vi "Main axis motion_單步.vi"(0 "Tacc/Tdec":u32, 1 "axis":u8, 2 "VL/VH":i32, 3 "Position":i32, 4 "¶bemg+":i32, 5 "¶bemg -":i32, 6 "Axis motion function":T1, 7 "error in (no error)":errorcluster, 8 "CK mode":enum16{"motion status", "current position"}(ring), 9 "Ref. data":refnum<vi>, 11 "是否要看軟體極限?":bool) -> (15 "error_code":u32, 17 "current_posi":i32, 19 "error out":errorcluster)   [LabVIEW 2014]
uses:
  axis motion function.ctl
panel:
  in  "error in (no error) 2":errorcluster
  in  "Cluster":T2
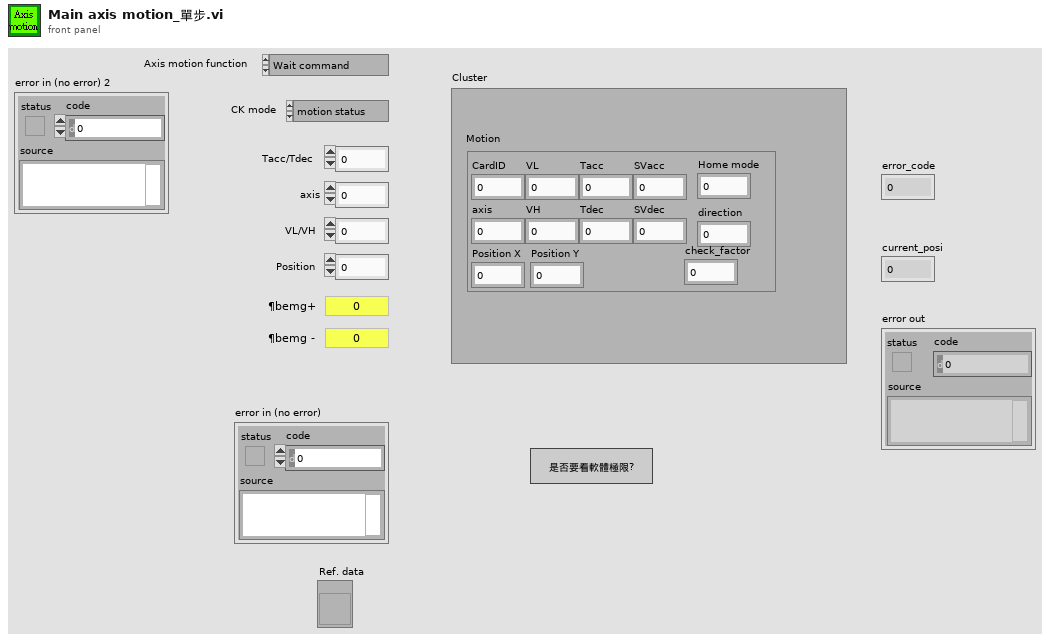
[diagram p1: front panel]
types:
  T1 = typedef "axis motion function.ctl" = enum16{"Wait command", "Axis_S motion", "Axis_P motion", "Axis_Motion_Satus_CK", "Axis _S position CK", "Axis_P position CK", "finish", "error"}
  T2 = cluster{"Motion":cluster{"CardID":u8, "axis":u8, "VL":i32, "VH":i32, "Tacc":u32, "Tdec":u32, "SVacc":u32, "SVdec":u32, "Position X":i32, "Position Y":i32, "Home mode":u8, "direction":u8, "check_factor":u8}}
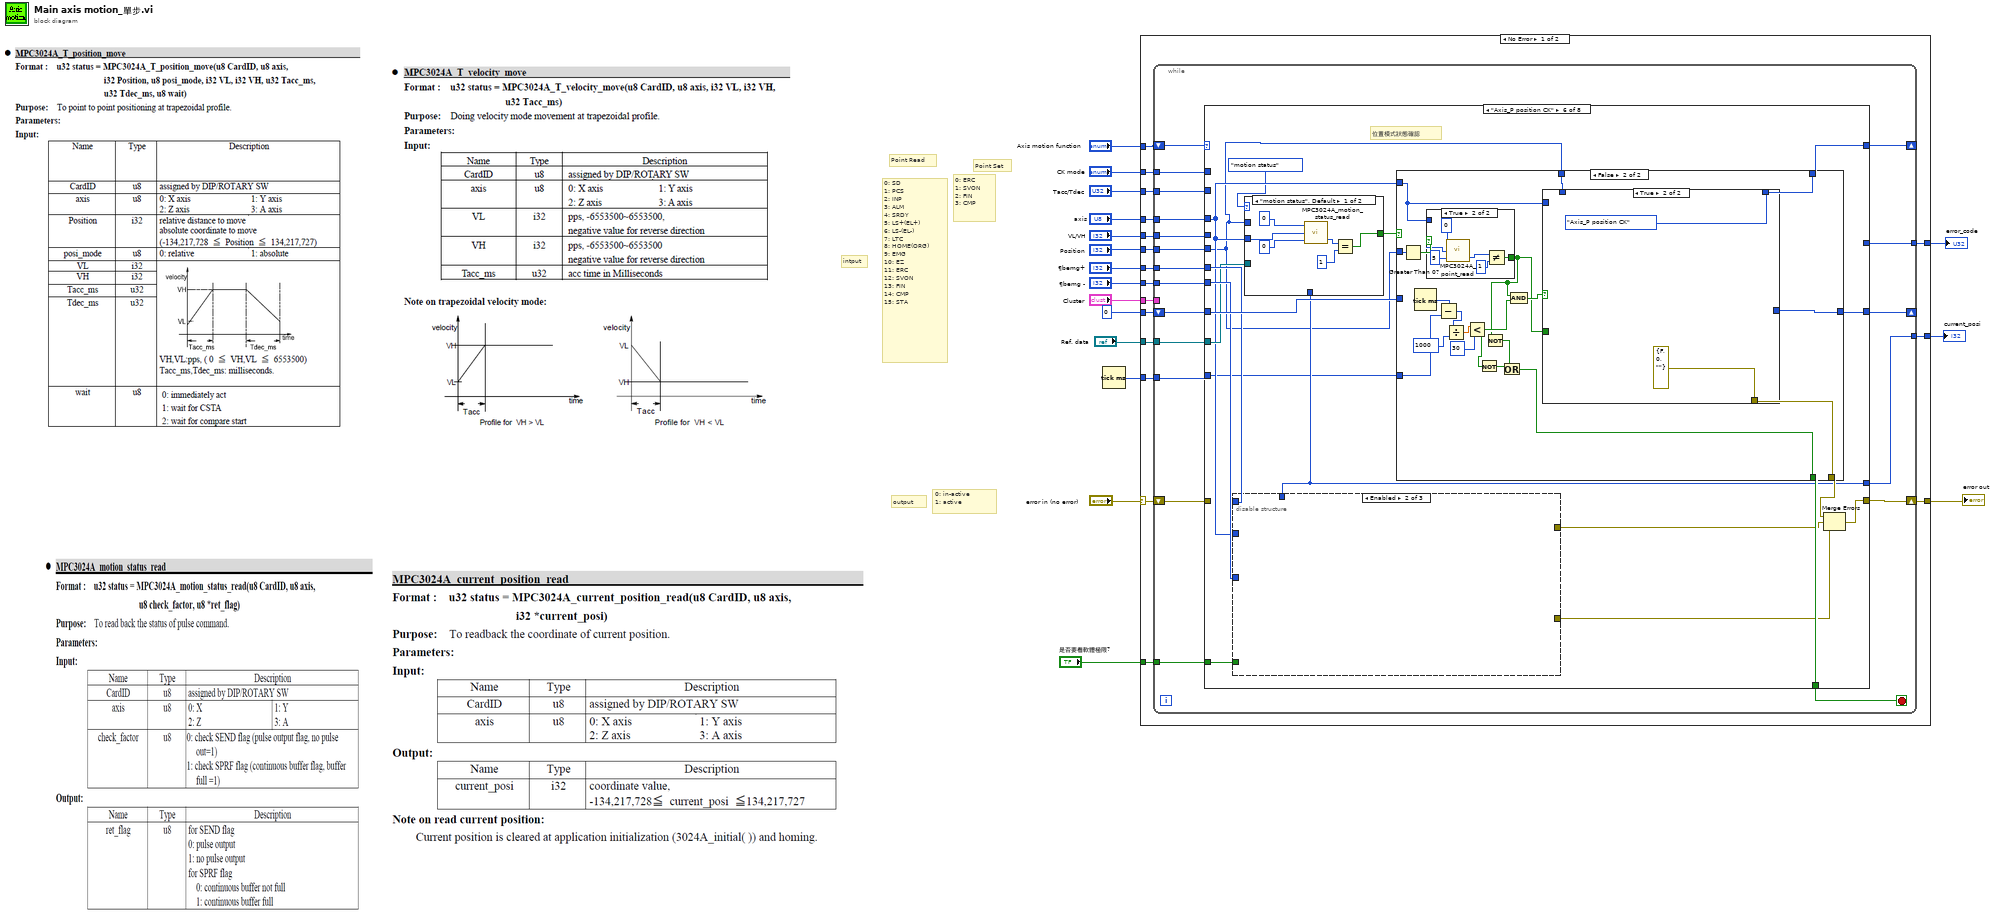
[diagram p0: block diagram]
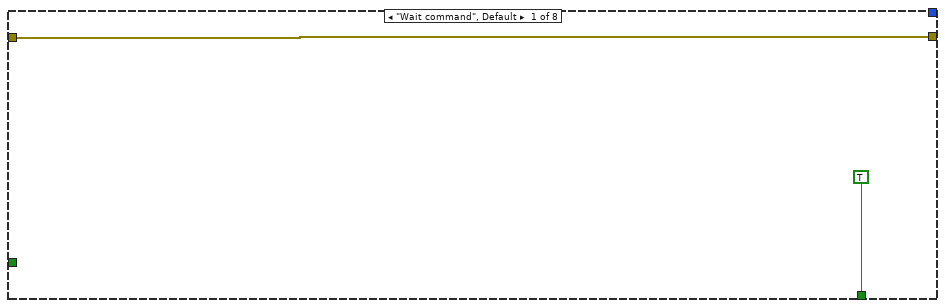
[diagram p2: hidden frame]
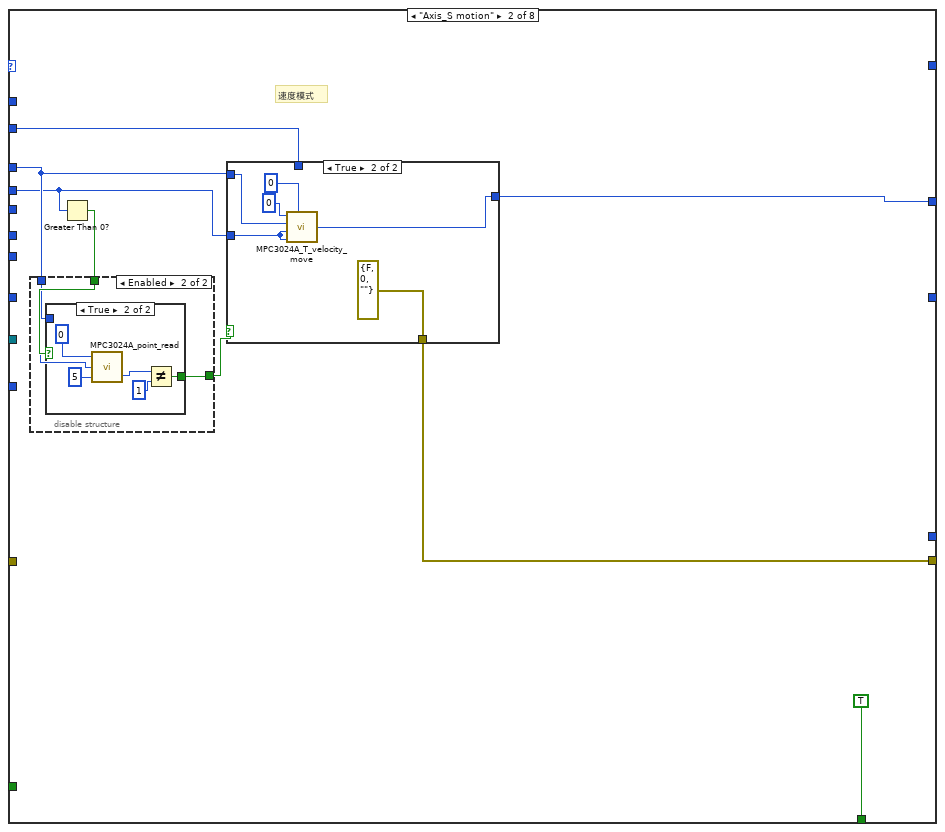
[diagram p3: hidden frame]
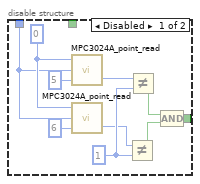
[diagram p4: hidden frame]
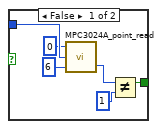
[diagram p5: hidden frame]
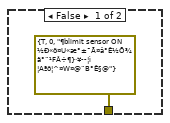
[diagram p6: hidden frame]
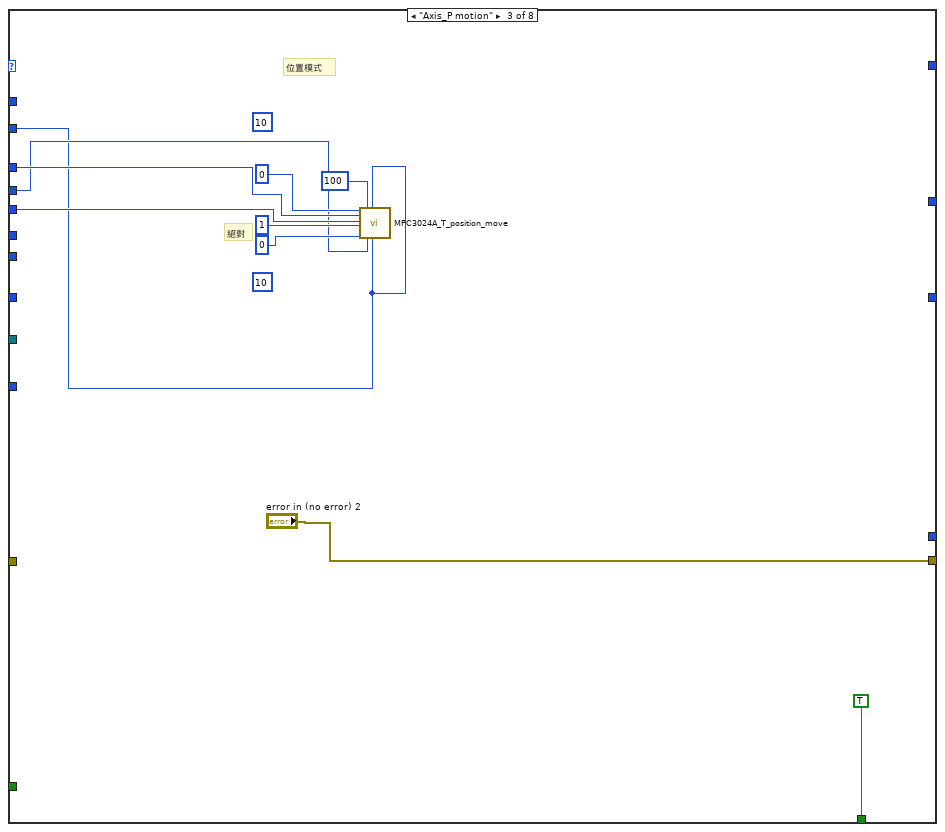
[diagram p7: hidden frame]
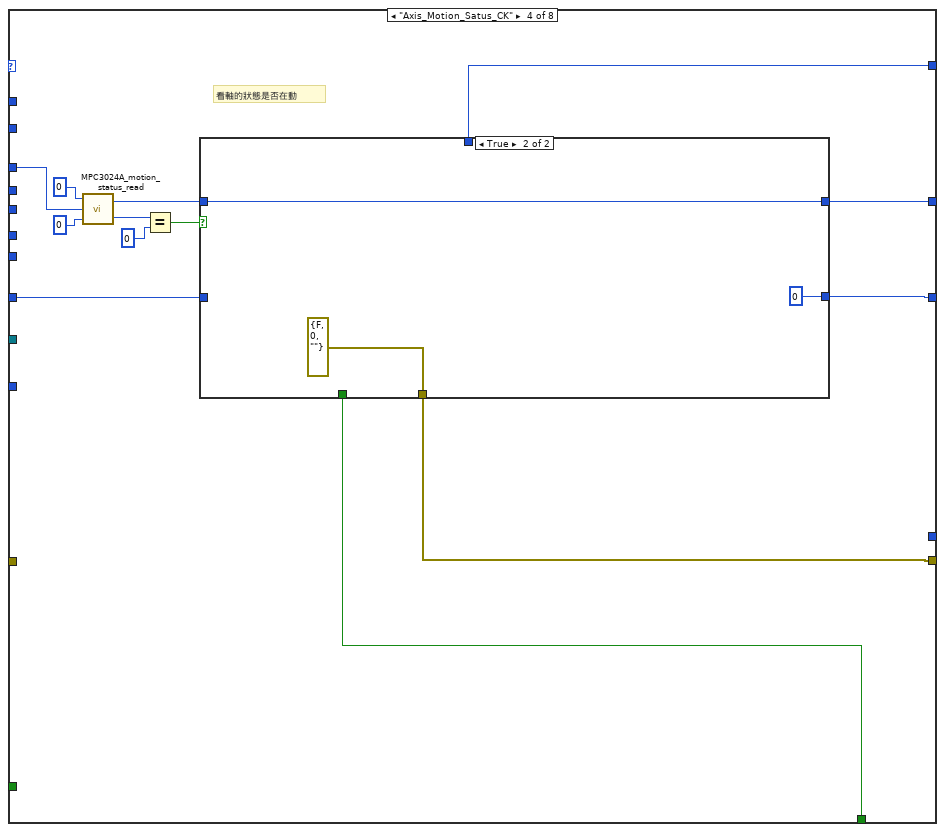
[diagram p8: hidden frame]
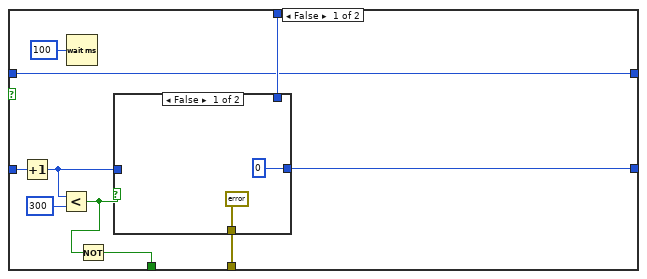
[diagram p9: hidden frame]
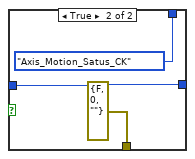
[diagram p10: hidden frame]
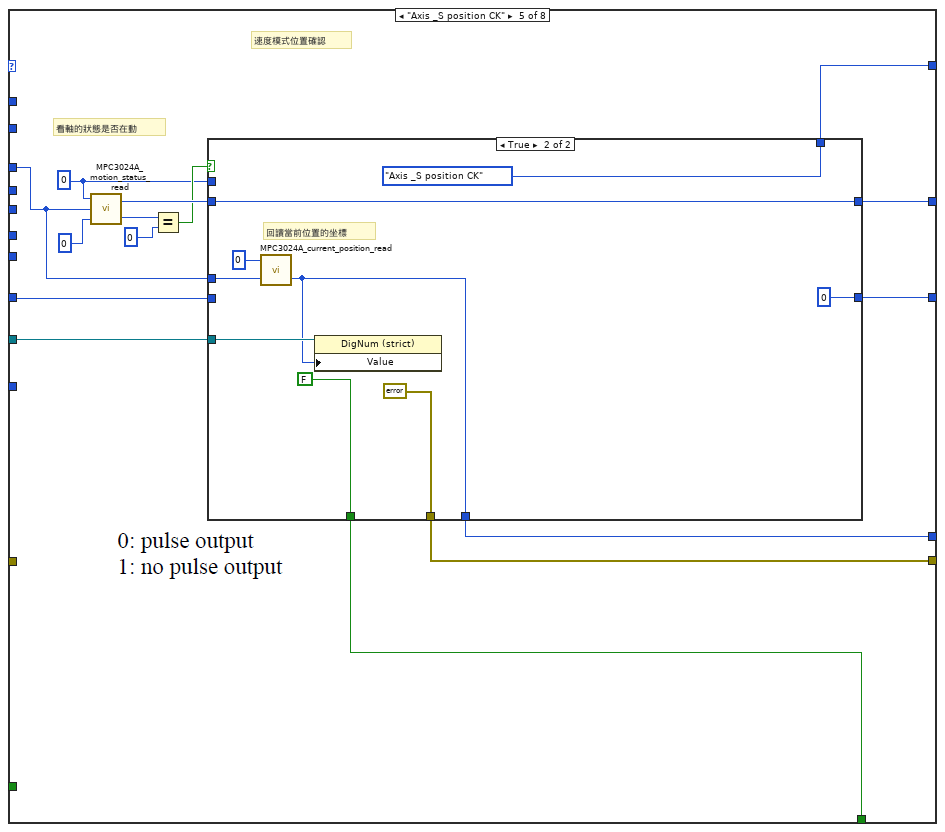
[diagram p11: hidden frame]
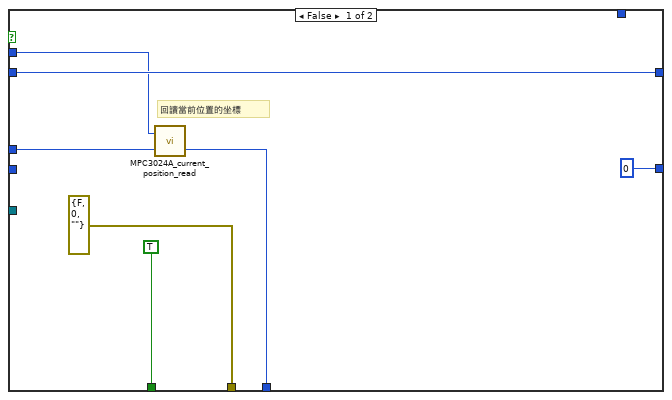
[diagram p12: hidden frame]
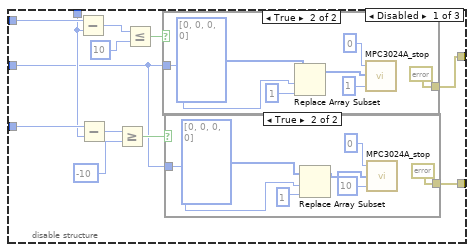
[diagram p13: hidden frame]
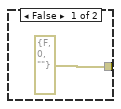
[diagram p14: hidden frame]
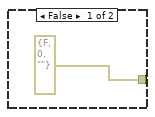
[diagram p15: hidden frame]
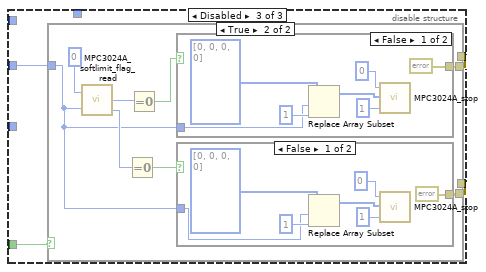
[diagram p16: hidden frame]
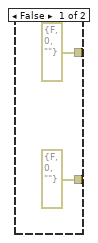
[diagram p17: hidden frame]
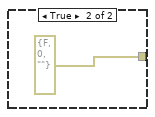
[diagram p18: hidden frame]
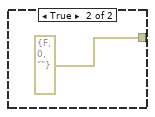
[diagram p19: hidden frame]
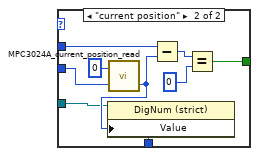
[diagram p20: hidden frame]
diagram:
  # "0: in-active   \n1: active"
  # "output"
  # "intput"
  # "Point Set"
  # "0: ERC   \n1: SVON  \n2: FIN\n3: CMP"
  # "Point Read"
  # "0: SD   \n1: PCS  \n2: INP\n3: ALM\n4: SRDY\n5: LS+(EL+)\n6: LS-(EL-)\n7: LTC\n8: HOME(ORG)\n9: EMG\n10: EZ\n11: ERC\n12: SVON\n13: FIN\n14: CMP\n15: STA"
  n1 = Tick Count (ms)() -> (millisecond timer value=w1:u32)
  n2 = case shown="No Error" "error in (no error)" {
    selector: "error in (no error)" -> [w33 w325]
    tunnel: "Axis motion function" -> [w31 _]
    tunnel: [w34 w325] -> w17
    tunnel: 0 -> [w26 _]
    tunnel: "Cluster" -> [w32 _]
    tunnel: "axis" -> [w30 _]
    tunnel: "VL/VH" -> [w29 _]
    tunnel: "Position" -> [w28 _]
    tunnel: "Tacc/Tdec" -> [w27 _]
    tunnel: [w25 _] -> w8
    tunnel: "CK mode" -> [w24 _]
    tunnel: [w23 _] -> w6
    tunnel: "¶bemg+" -> [w22 _]
    tunnel: "¶bemg -" -> [w21 _]
    tunnel: "Ref. data" -> [w20 _]
    tunnel: "是否要看軟體極限?" -> [w19 _]
    tunnel: w1 -> [w18 _]
    frame No Error {
      n3 = while {
        shift-right: [w45] -> w34
        shift-left: w33 -> [w43]
        tunnel: w32 -> [_]
        shift-right: [w52] -> _
        shift-left: w31 -> [w53]
        tunnel: w30 -> [w51]
        tunnel: w29 -> [w50]
        tunnel: w28 -> [w49]
        tunnel: w27 -> [w48]
        shift-right: [w46] -> _
        shift-left: w26 -> [w47]
        tunnel: [w42] -> w25
        tunnel: w24 -> [w41]
        tunnel: [w40] -> w23
        tunnel: w22 -> [w39]
        tunnel: w21 -> [w38]
        tunnel: w20 -> [w37]
        tunnel: w19 -> [w36]
        tunnel: w18 -> [w35]
        stop <- w44 stop-if-true
        n4 = case shown="\"Axis_P position CK\"" w53 {
          tunnel: [_ _ _ w106 w138 w182 _ _] -> w52
          tunnel: w51 -> [_ w58 w99 w112 w140 w171 _ _]
          tunnel: w50 -> [_ w57 w98 _ _ _ _ _]
          tunnel: w49 -> [_ _ w100 _ _ w168 _ _]
          tunnel: w48 -> [_ w59 w97 _ _ _ _ _]
          tunnel: w47 -> [_ _ _ w109 w150 w185 w320 w323]
          tunnel: [_ _ _ w110 w148 w184 w320 w323] -> w46
          tunnel: [w55 w61 "error in (no error) 2" w108 w151 w179 w321 w324] -> w45
          tunnel: [TRUE TRUE TRUE w111 w149 w183 _ TRUE] -> w44
          tunnel: w43 -> [w55 _ _ _ _ _ w321 w324]
          tunnel: [_ w60 _ w107 w147 _ _ _] -> w42
          tunnel: w41 -> [_ _ _ _ _ _ _ _]
          tunnel: [_ _ _ _ w139 w175 _ _] -> w40
          tunnel: w39 -> [_ _ _ _ _ w180 _ _]
          tunnel: w38 -> [_ _ _ _ _ w176 _ _]
          tunnel: w37 -> [_ _ _ _ w137 w173 _ _]
          tunnel: w36 -> [_ _ _ _ _ w172 _ _]
          tunnel: w35 -> [_ _ _ _ _ w170 _ _]
          frame "Wait command", Default {
          }
          frame "Axis_S motion" {
            # "速度模式"
            n5 = Greater Than 0?(x=w57) -> (x > 0?=w56:bool)
            n6 = disable-structure shown="Enabled" {
              disable-tunnel: [w65 w74] -> w62
              disable-tunnel: w58 -> [w64 w75]
              disable-tunnel: w56 -> [_ w76]
              frame Disabled {
                w66 = u8 0 ("axis")
                w71 = u8 1 ("y")
                n7 = call "MPC3024A_point_read.vi"("check_factor"=u8 5, "axis"=w64, "CardID"=w66) -> ("state"=w70:u8)  [unwired: 1 out]
                n8 = call "MPC3024A_point_read.vi"("check_factor"=u8 6, "axis"=w64, "CardID"=w66) -> ("state"=w69:u8)  [unwired: 1 out]
                n9 = Not Equal?(x=w69, y=w71) -> (x != y?=w68:bool)
                n10 = Not Equal?(x=w70, y=w71) -> (x != y?=w67:bool)
                n11 = Compound Arithmetic op=AND(w67, w68) -> (w65:bool)
              }
              frame Enabled {
                n12 = case shown="True" w76 {
                  tunnel: w75 -> [w81 w86]
                  tunnel: [w77 w83] -> w74
                  frame False {
                    n13 = call "MPC3024A_point_read.vi"("check_factor"=u8 6, "axis"=w81, "CardID"=u8 0) -> ("state"=w78:u8)  [unwired: 1 out]
                    n14 = Not Equal?(x=w78, y=u8 1) -> (x != y?=w77:bool)
                  }
                  frame True {
                    n15 = call "MPC3024A_point_read.vi"("check_factor"=u8 5, "axis"=w86, "CardID"=u8 0 ("axis")) -> ("state"=w85:u8)  [unwired: 1 out]
                    n16 = Not Equal?(x=w85, y=u8 1) -> (x != y?=w83:bool)
                  }
                }
              }
            }
            n17 = case shown="True" w62 {
              tunnel: [_ w95] -> w60
              tunnel: [errorcluster {"status"=TRUE, "code"=0, "source"="¶blimit sensor ON ½Ð«ö¤U«æ°±¯Ã¤â°Ê½Õ¾ã°¨¹FÂ÷¶}·¥­­¦ì ¦Aªð¦^¤W¤@¨B°Ê§@"} ("error in (no error)") errorcluster {"status"=FALSE, "code"=0, "source"=""} ("error in (no error)")] -> w61
              tunnel: w59 -> [_ _]
              tunnel: w58 -> [_ w92]
              tunnel: w57 -> [_ w91]
              frame False {
              }
              frame True {
                n18 = call "MPC3024A_T_velocity_move.vi"("CardID"=u8 0, "axis"=w92, "VL"=w91, "VH"=w91, "Tacc_ms"=u32 0) -> ("error_code"=w95:u32)
              }
            }
          }
          frame "Axis_P motion" {
            (unwired) u32 10 ("Tdec_ms")
            (unwired) u32 10 ("Tacc_ms")
            # "位置模式"
            # "絕對"
            n19 = call "MPC3024A_T_position_move.vi"("CardID"=u8 0, "axis"=w99, "Position"=w100, "posi_mode"=u8 1, "wait"=u8 0, "VL"=100, "VH"=w98, "Tacc_ms"=w97, "Tdec_ms"=w97) -> ()  [unwired: 10 in, 1 out]
          }
          frame "Axis_Motion_Satus_CK" {
            # "看軸的狀態是否在動"
            n20 = call "MPC3024A_motion_status_read.vi"("check_factor"=u8 0, "axis"=w112, "CardID"=u8 0) -> ("ret_fig"=w115:u8, "error_code"=w114:u32)
            n21 = Equal?(x=w115, y=u8 0) -> (x = y?=w113:bool)
            n22 = case shown="True" w113 {
              tunnel: [w124 errorcluster {"status"=FALSE, "code"=0, "source"=""} ("error in (no error)")] -> w108
              tunnel: w109 -> [w119 _]
              tunnel: [w126 _] -> w111
              tunnel: [w123 _] -> w106
              tunnel: [w122 0] -> w110
              tunnel: [w120 w134] -> w107
              tunnel: w114 -> [w120 w134]
              frame False {
                n23 = Increment(x=w119) -> (x+1=w121:i32)
                n24 = Less?(x=w121, y=300) -> (x < y?=w125:bool)
                n25 = Wait (ms)(milliseconds to wait=u32 100) -> ()  [unwired: 1 out]
                n26 = Not(x=w125) -> (.not. x?=w126:bool)
                n27 = case shown="False" w125 {
                  tunnel: [errorcluster {"status"=TRUE, "code"=0, "source"="軸沒輸出移動脈波"} ("error in (no error)") errorcluster {"status"=FALSE, "code"=0, "source"=""} ("error in (no error)")] -> w124
                  tunnel: [_ axis_motion_function."Axis_Motion_Satus_CK" ("Axis motion function")] -> w123
                  tunnel: [0 w131] -> w122
                  tunnel: w121 -> [_ w131]
                  frame False {
                  }
                  frame True {
                  }
                }
              }
              frame True {
              }
            }
          }
          frame "Axis _S position CK" {
            w141 = u8 0 ("CardID")
            # "速度模式位置確認"
            # "看軸的狀態是否在動"
            n28 = call "MPC3024A_motion_status_read.vi"("check_factor"=u8 0, "axis"=w140, "CardID"=w141) -> ("ret_fig"=w144:u8, "error_code"=w143:u32)
            n29 = Equal?(x=w144, y=u8 0) -> (x = y?=w142:bool)
            n30 = case shown="True" w142 {
              tunnel: [errorcluster {"status"=FALSE, "code"=0, "source"=""} ("error in (no error)") errorcluster {"status"=FALSE, "code"=0, "source"=""} ("error in (no error)")] -> w151
              tunnel: w150 -> [_ _]
              tunnel: [TRUE FALSE] -> w149
              tunnel: [_ axis_motion_function."Axis _S position CK" ("Axis motion function")] -> w138
              tunnel: [0 0] -> w148
              tunnel: [w157 w165] -> w147
              tunnel: w143 -> [w157 w165]
              tunnel: w141 -> [w155 _]
              tunnel: w140 -> [w156 w164]
              tunnel: [w152 w161] -> w139
              tunnel: w137 -> [_ w162]
              frame False {
                # "回讀當前位置的坐標"
                n31 = call "MPC3024A_current_position_read.vi"("axis"=w156, "CardID"=w155) -> ("current_posi"=w152:i32)  [unwired: 1 out]
              }
              frame True {
                # "回讀當前位置的坐標"
                n32 = call "MPC3024A_current_position_read.vi"("axis"=w164, "CardID"=u8 0) -> ("current_posi"=w161:i32)  [unwired: 1 out]
                n33 = property class="DigNum (strict)"(reference=w162, "Value"=w161) -> ()  [unwired: 1 in, 2 out]
              }
            }
          }
          frame "Axis_P position CK" {
            # "位置模式狀態確認"
            n34 = case shown="\"motion status\", Default" enum16{"motion status", "current position"}."motion status" ("CK mode") {
              tunnel: [w245 w254] -> w181
              tunnel: w171 -> [w244 w253]
              tunnel: w168 -> [_ w252]
              tunnel: [_ w251] -> w175
              tunnel: w173 -> [_ w250]
              frame "motion status", Default {
                n35 = call "MPC3024A_motion_status_read.vi"("check_factor"=u8 0, "axis"=w244, "CardID"=u8 0) -> ("ret_fig"=w246:u8)  [unwired: 1 out]
                n36 = Equal?(x=w246, y=u8 1) -> (x = y?=w245:bool)
              }
              frame "current position" {
                n37 = call "MPC3024A_current_position_read.vi"("axis"=w253, "CardID"=u8 0) -> ("current_posi"=w251:i32)  [unwired: 1 out]
                n38 = property class="DigNum (strict)"(reference=w250, "Value"=w251) -> ()  [unwired: 1 in, 2 out]
                n39 = Subtract(x=w252, y=w251) -> (x-y=w256:i32)
                n40 = Equal?(x=w256, y=0) -> (x = y?=w254:bool)
              }
            }
            n41 = disable-structure shown="Enabled" {
              disable-tunnel: w180 -> [w197 _ _]
              disable-tunnel: [w193 _ w217] -> w177
              disable-tunnel: w176 -> [w190 _ _]
              disable-tunnel: w175 -> [w189 _ _]
              disable-tunnel: [w188 _ w216] -> w174
              disable-tunnel: w171 -> [w186 _ w214]
              disable-tunnel: w172 -> [_ _ w215]
              frame Disabled {
                n42 = Subtract(x=w197, y=w189) -> (x-y=w196:i32)
                n43 = Subtract(x=w190, y=w189) -> (x-y=w187:i32)
                n44 = Greater Or Equal?(x=w187, y=-10) -> (x >= y?=w192:bool)
                n45 = Less Or Equal?(x=w196, y=10) -> (x <= y?=w194:bool)
                n46 = case shown="True" w194 {
                  tunnel: [errorcluster {"status"=FALSE, "code"=0, "source"=""} ("error in (no error)") errorcluster {"status"=TRUE, "code"=0, "source"="軸接近後軟體極限"} ("error in (no error)")] -> w193
                  tunnel: w186 -> [_ w207]
                  frame False {
                  }
                  frame True {
                    n47 = Replace Array Subset(array=i32[] [0, 0, 0, 0], new element=1 ("new element/subarray"), index=w207) -> (w208:i32[])
                    n48 = call "MPC3024A_stop.vi"("Tdec_ms"=u32 1, "axis[4]"=w208, "CardID"=u8 0) -> ()  [unwired: 1 out]
                  }
                }
                n49 = case shown="True" w192 {
                  tunnel: [errorcluster {"status"=FALSE, "code"=0, "source"=""} ("error in (no error)") errorcluster {"status"=TRUE, "code"=0, "source"="軸接近前軟體極限"} ("error in (no error)")] -> w188
                  tunnel: w186 -> [_ w199]
                  frame False {
                  }
                  frame True {
                    n50 = Replace Array Subset(array=i32[] [0, 0, 0, 0], new element=1 ("new element/subarray"), index=w199) -> (w202:i32[])
                    n51 = call "MPC3024A_stop.vi"("Tdec_ms"=u32 10, "axis[4]"=w202, "CardID"=u8 0) -> ()  [unwired: 1 out]
                  }
                }
              }
              frame Enabled {
              }
              frame Disabled {
                n52 = case shown="True" w215 {
                  tunnel: [errorcluster {"status"=FALSE, "code"=0, "source"=""} ("error in (no error)") w223] -> w217
                  tunnel: [errorcluster {"status"=FALSE, "code"=0, "source"=""} ("error in (no error)") w222] -> w216
                  tunnel: w214 -> [_ w220]
                  frame False {
                  }
                  frame True {
                    n53 = call "MPC3024A_softlimit_flag_read.vi"("CardID"=u8 0, "axis"=w220) -> ("P_limit_flag"=w226:u8, "N_limit_flag"=w225:u8)  [unwired: 1 out]
                    n54 = Equal To 0?(x=w225) -> (x = 0?=w221:bool)
                    n55 = Equal To 0?(x=w226) -> (x = 0?=w224:bool)
                    n56 = case shown="False" w224 {
                      tunnel: [errorcluster {"status"=TRUE, "code"=0, "source"="軸接近前軟體極限"} ("error in (no error)") errorcluster {"status"=FALSE, "code"=0, "source"=""} ("error in (no error)")] -> w223
                      tunnel: w220 -> [w236 _]
                      frame False {
                        n57 = Replace Array Subset(array=i32[] [0, 0, 0, 0], new element=1 ("new element/subarray"), index=w236) -> (w237:i32[])
                        n58 = call "MPC3024A_stop.vi"("Tdec_ms"=u32 1, "axis[4]"=w237, "CardID"=u8 0) -> ()  [unwired: 1 out]
                      }
                      frame True {
                      }
                    }
                    n59 = case shown="False" w221 {
                      tunnel: [errorcluster {"status"=TRUE, "code"=0, "source"="軸接近後軟體極限"} ("error in (no error)") errorcluster {"status"=FALSE, "code"=0, "source"=""} ("error in (no error)")] -> w222
                      tunnel: w220 -> [w228 _]
                      frame False {
                        n60 = Replace Array Subset(array=i32[] [0, 0, 0, 0], new element=1 ("new element/subarray"), index=w228) -> (w229:i32[])
                        n61 = call "MPC3024A_stop.vi"("Tdec_ms"=u32 1, "axis[4]"=w229, "CardID"=u8 0) -> ()  [unwired: 1 out]
                      }
                      frame True {
                      }
                    }
                  }
                }
              }
            }
            n62 = case shown="False" w181 {
              selector: w181 -> [w262 _]
              tunnel: w185 -> [_ _]
              tunnel: [_ w289] -> w184
              tunnel: [w267 w290] -> w178
              tunnel: [w262 w274] -> w183
              tunnel: [axis_motion_function."finish" ("Axis motion function") w291] -> w182
              tunnel: w168 -> [_ w287]
              tunnel: w171 -> [w266 w275]
              tunnel: w170 -> [_ w285]
              tunnel: w168 -> [w265 w279]
              frame True {
                # "+-10pulse"
                n63 = call "MPC3024A_current_position_read.vi"("axis"=w266, "CardID"=u8 0) -> ("current_posi"=w263:i32)  [unwired: 1 out]
                n64 = Subtract(x=w265, y=w263) -> (x-y=w261:i32)
                n65 = In Range and Coerce(upper limit=10.0, x=w261, lower limit=10.0 ("upper limit")) -> (In Range?=w258:bool)  [unwired: 1 out]
                n66 = disable-structure shown="Disabled" {
                  disable-tunnel: [w270 _] -> w267
                  disable-tunnel: w258 -> [w269 _]
                  frame Disabled {
                    n67 = case shown="False" w269 {
                      tunnel: [errorcluster {"status"=TRUE, "code"=0, "source"="未移到指定位置"} ("error in (no error)") errorcluster {"status"=FALSE, "code"=0, "source"=""} ("error in (no error)")] -> w270
                      frame False {
                      }
                      frame True {
                      }
                    }
                  }
                  frame Enabled {
                  }
                }
              }
              frame False {
                n68 = Greater Than 0?(x=w287) -> (x > 0?=w288:bool)
                n69 = Tick Count (ms)() -> (millisecond timer value=w286:u32)
                n70 = case shown="True" w288 {
                  tunnel: w275 -> [w296 w301]
                  tunnel: [w292 w298] -> w278
                  frame False {
                    n71 = call "MPC3024A_point_read.vi"("check_factor"=u8 6, "axis"=w296, "CardID"=u8 0) -> ("state"=w293:u8)  [unwired: 1 out]
                    n72 = Not Equal?(x=w293, y=u8 1) -> (x != y?=w292:bool)
                  }
                  frame True {
                    n73 = call "MPC3024A_point_read.vi"("check_factor"=u8 5, "axis"=w301, "CardID"=u8 0 ("axis")) -> ("state"=w300:u8)  [unwired: 1 out]
                    n74 = Not Equal?(x=w300, y=u8 1) -> (x != y?=w298:bool)
                  }
                }
                n75 = Subtract(x=w286, y=w285) -> (x-y=w284:u32)
                n76 = Divide(x=w284, y=u32 1000) -> (x/y=w273:dbl)
                n77 = Less?(x=w273, y=30) -> (x < y?=w281:bool)
                n78 = Not(x=w281) -> (.not. x?=w276:bool)
                n79 = Not(x=w278) -> (.not. x?=w277:bool)
                n80 = Or(x=w276, y=w277) -> (x .or. y?=w274:bool)
                n81 = And(x=w278, y=w281) -> (x .and. y?=w280:bool)
                n82 = case shown="True" w280 {
                  tunnel: [0 _] -> w289
                  tunnel: [w314 errorcluster {"status"=FALSE, "code"=0, "source"=""} ("error in (no error)")] -> w290
                  tunnel: [w312 axis_motion_function."Axis_P position CK" ("Axis motion function")] -> w291
                  tunnel: w278 -> [w311 _]
                  tunnel: w275 -> [w308 _]
                  tunnel: w279 -> [_ _]
                  frame False {
                    n83 = Not(x=w311) -> (.not. x?=w310:bool)
                    n84 = Replace Array Subset(array=i32[] [0, 0, 0, 0], new element=1 ("new element/subarray"), index=w308) -> (w304:i32[])
                    n85 = call "MPC3024A_stop.vi"("Tdec_ms"=u32 1, "axis[4]"=w304, "CardID"=u8 0) -> ()  [unwired: 1 out]
                    n86 = case shown="False" w310 {
                      tunnel: [errorcluster {"status"=TRUE, "code"=0, "source"="動作超時"} ("error in (no error)") errorcluster {"status"=TRUE, "code"=0, "source"="碰極限"} ("error in (no error)")] -> w314
                      frame False {
                      }
                      frame True {
                      }
                    }
                    n87 = disable-structure shown="Enabled" {
                      disable-tunnel: [axis_motion_function."error" ("Axis motion function")] -> w312
                      frame Enabled {
                      }
                    }
                  }
                  frame True {
                  }
                }
              }
            }
            n88 = Merge Errors(w178, w177, w174) -> (w179:errorcluster)
          }
          frame "finish" {
          }
          frame "error" {
          }
        }
      }
    }
    frame Error {
    }
  }
  "error out" <- w17
  "current_posi" <- w6
  "error_code" <- w8
